vi "Edge-Edge distance.vi"(3 "Edge 2 start point":sgl[](array[numeric]), 4 "Edge 2 (not unit)":sgl[](array[numeric]), 5 "Edge 1 start point":sgl[](array[numeric]), 6 "Edge 1 (not unit)":sgl[](array[numeric])) -> (0 "Include":bool, 1 "Distance^2":sgl, 2 "Distance vector":sgl[](array[numeric]))   [LabVIEW 2018]
panel:
  # "PN 13/01/2015"
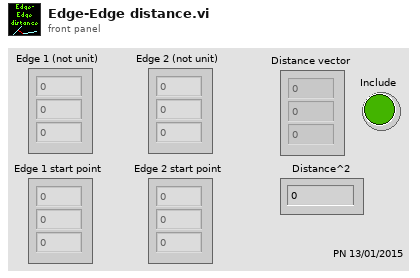
[diagram p1: front panel]
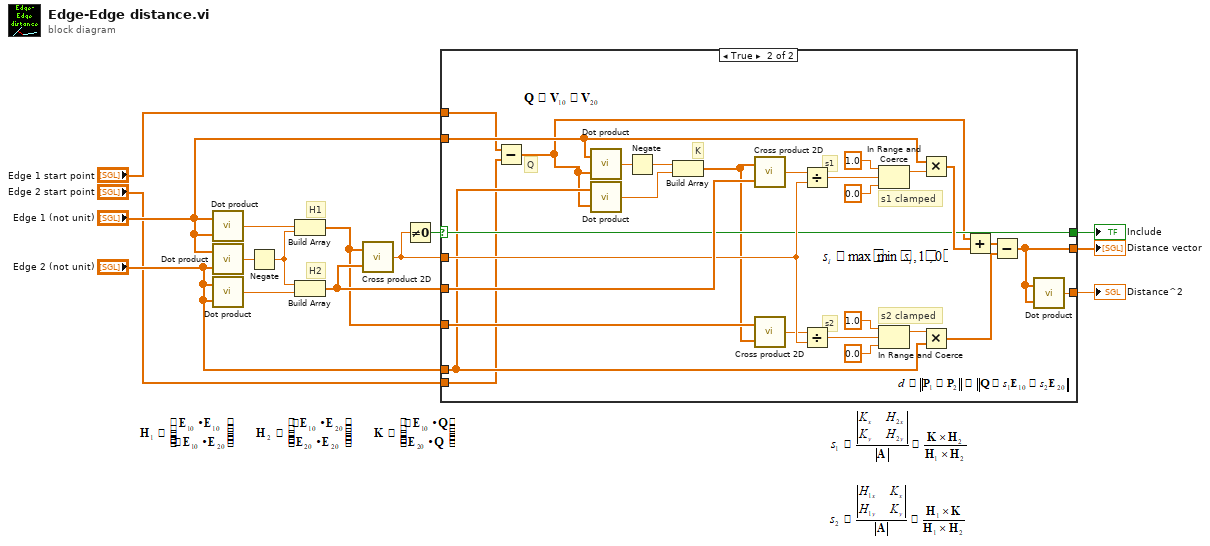
[diagram p0: block diagram]
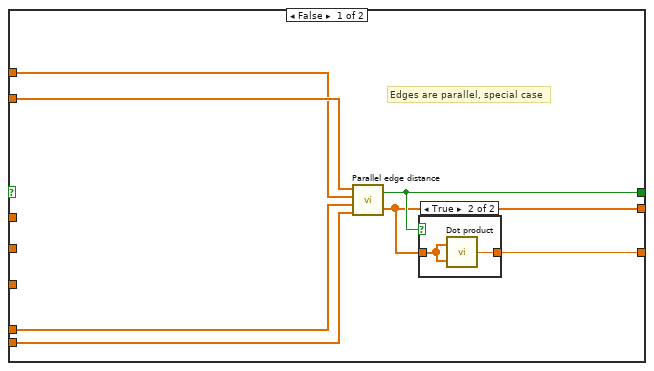
[diagram p2: hidden frame]
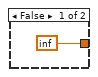
[diagram p3: hidden frame]
diagram:
  # "H2"
  # "H1"
  n1 = call "Dot product.vi"("B"="Edge 1 (not unit)", "A"="Edge 1 (not unit)") -> ("A . B"=w14:sgl)
  n2 = call "Dot product.vi"("B"="Edge 2 (not unit)", "A"="Edge 1 (not unit)") -> ("A . B"=w15:sgl)
  n3 = call "Dot product.vi"("B"="Edge 2 (not unit)", "A"="Edge 2 (not unit)") -> ("A . B"=w12:sgl)
  n4 = Negate(x=w15) -> (-x=w13:sgl)
  n5 = Build Array(w14, w13) -> (w10:sgl[])
  n6 = Build Array(w13, w12) -> (w11:sgl[])
  n7 = call "Cross product 2D.vi"("B"=w11, "A"=w10) -> ("A X B"=w7:sgl)
  n8 = Not Equal To 0?(x=w7) -> (x != 0?=w6:bool)
  n9 = case shown="True" w6 {
    selector: w6 -> [_ w37]
    tunnel: w11 -> [_ w53]
    tunnel: w10 -> [_ w52]
    tunnel: "Edge 1 (not unit)" -> [w22 w31]
    tunnel: "Edge 2 (not unit)" -> [w21 w29]
    tunnel: [w17 w35] -> w3
    tunnel: w7 -> [_ w46]
    tunnel: "Edge 1 start point" -> [w20 w28]
    tunnel: "Edge 2 start point" -> [w19 w27]
    tunnel: [w18 w37] -> w2
    tunnel: [w16 w36] -> w1
    frame False {
      # "Edges are parallel, special case"
      n10 = call "Parallel edge distance.vi"("Edge 2 start point"=w19, "Edge 2 (not unit)"=w21, "Edge 1 start point"=w20, "Edge 1 (not unit)"=w22) -> ("Distance vector"=w17:sgl[], "Projections overlap"=w18:bool)
      n11 = case shown="True" w18 {
        tunnel: w17 -> [_ w25]
        tunnel: [sgl inf w24] -> w16
        frame False {
        }
        frame True {
          n12 = call "Dot product.vi"("B"=w25, "A"=w25) -> ("A . B"=w24:sgl)
        }
      }
    }
    frame True {
      # "Q"
      # "K"
      # "s2 clamped"
      # "s1 clamped"
      # "s2"
      # "s1"
      n13 = Subtract(x=w28, y=w27) -> (x-y=w26:sgl[])
      n14 = call "Dot product.vi"("B"=w26, "A"=w31) -> ("A . B"=w33:sgl)
      n15 = call "Dot product.vi"("B"=w26, "A"=w29) -> ("A . B"=w30:sgl)
      n16 = Negate(x=w33) -> (-x=w34:sgl)
      n17 = Build Array(w34, w30) -> (w32:sgl[])
      n18 = call "Cross product 2D.vi"("B"=w53, "A"=w32) -> ("A X B"=w45:sgl)
      n19 = call "Cross product 2D.vi"("B"=w32, "A"=w52) -> ("A X B"=w44:sgl)
      n20 = Divide(x=w45, y=w46) -> (x/y=w41:sgl)
      n21 = Divide(x=w44, y=w46) -> (x/y=w38:sgl)
      n22 = In Range and Coerce(upper limit=sgl 1.0, x=w41, lower limit=sgl 0.0) -> (coerced(x)=w51:sgl)  [unwired: 1 out]
      n23 = In Range and Coerce(upper limit=sgl 1.0, x=w38, lower limit=sgl 0.0) -> (coerced(x)=w50:sgl)  [unwired: 1 out]
      n24 = Multiply(x=w31, y=w51) -> (x*y=w49:sgl[])
      n25 = Multiply(x=w50, y=w29) -> (x*y=w47:sgl[])
      n26 = Add(x=w26, y=w49) -> (x+y=w48:sgl[])
      n27 = Subtract(x=w48, y=w47) -> (x-y=w35:sgl[])
      n28 = call "Dot product.vi"("B"=w35, "A"=w35) -> ("A . B"=w36:sgl)
    }
  }
  "Distance vector" <- w3
  "Include" <- w2
  "Distance^2" <- w1
